vi "Polar Graph Drawer.vi"(8 "error in":errorcluster, 10 "Plot Right":dbl[](array[numeric]), 11 "Plot Left":dbl[](array[numeric])) -> (0 "error out":errorcluster, 3 "Polar Graph":cluster{dbl[], dbl[]}[](graph))   [LabVIEW 2025]
uses:
  <vilib>/Analysis/baseanly.llb/Mean (DBL).vi
  <vilib>/Analysis/NI_AALBase.lvlib
  <vilib>/gmath/NI_Gmath.lvlib
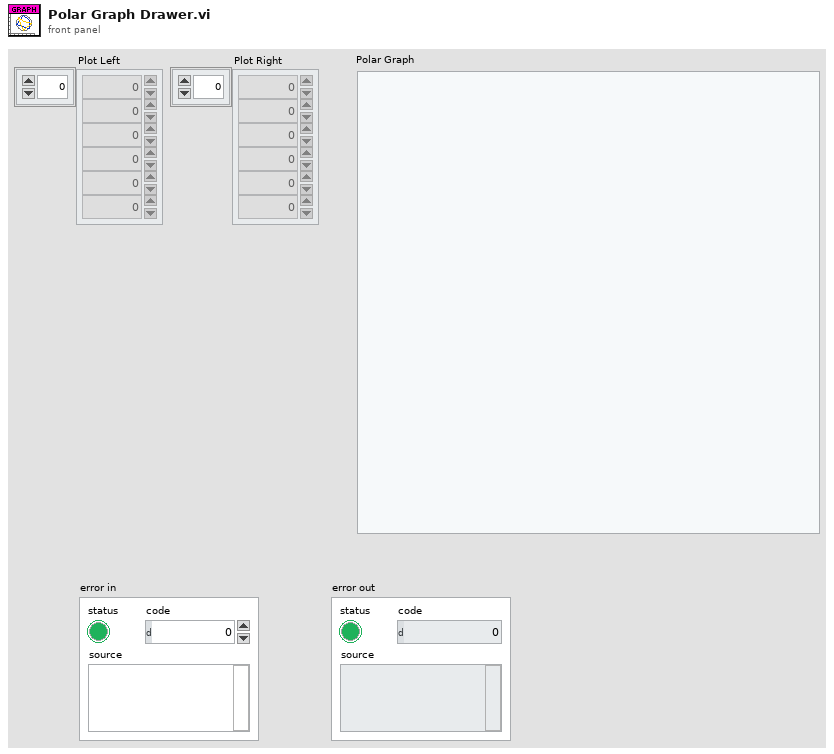
[diagram p1: front panel]
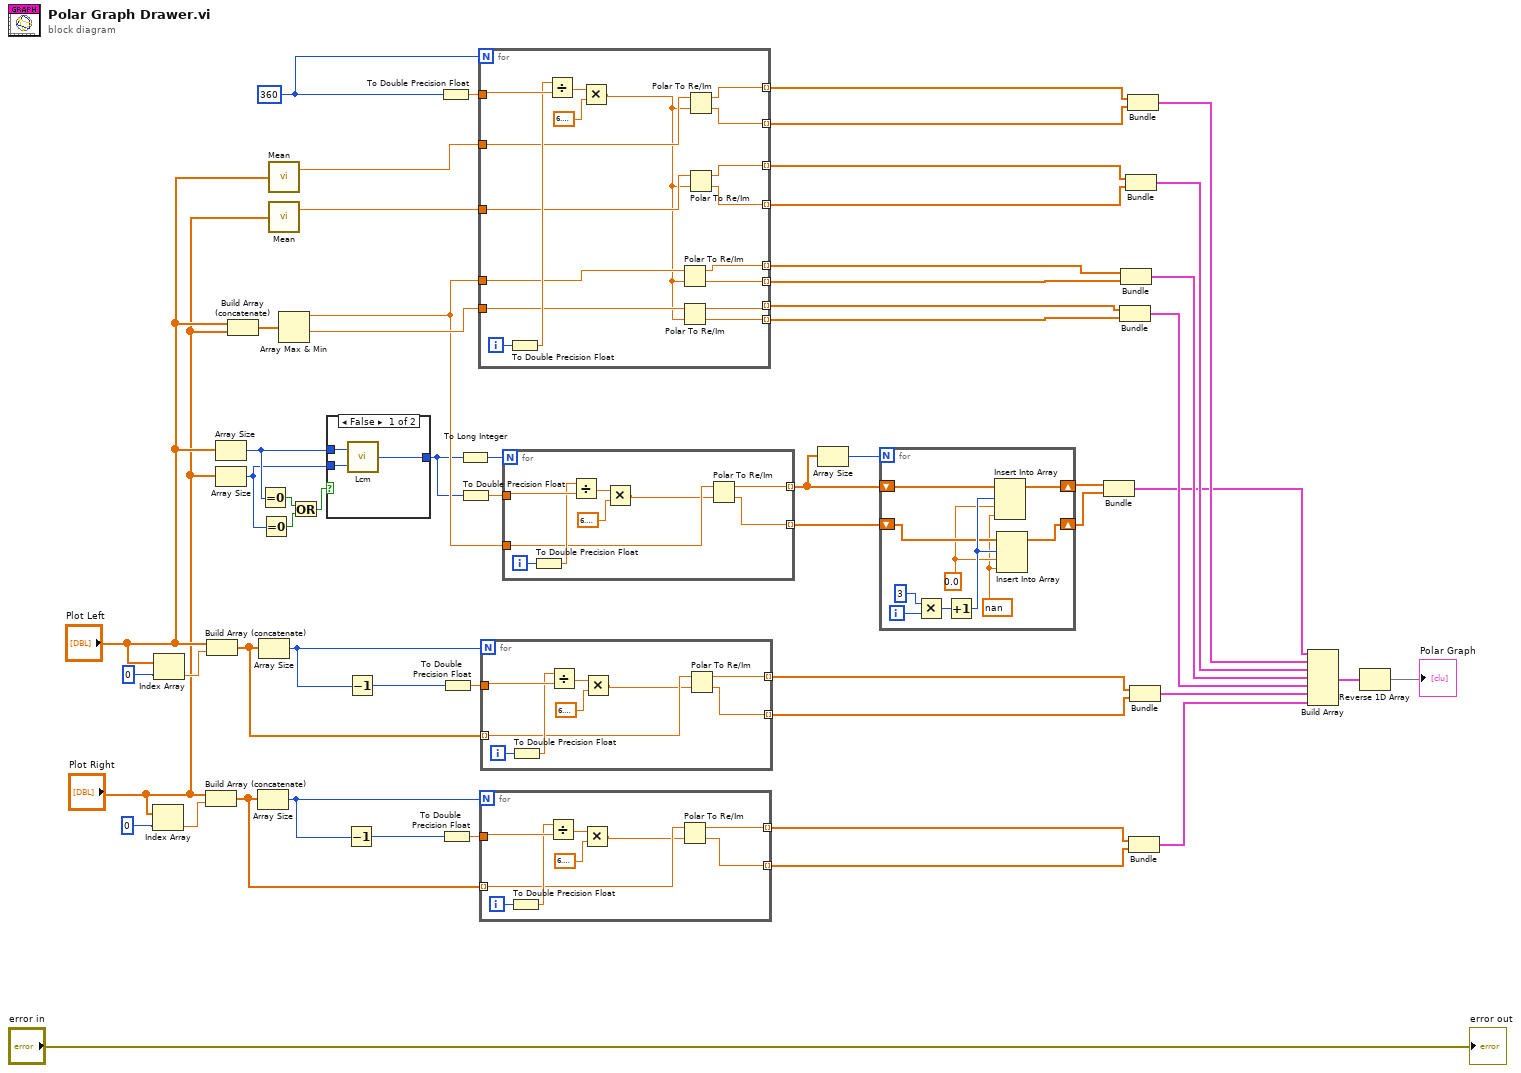
[diagram p0: block diagram]
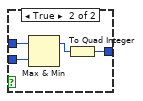
[diagram p2: hidden frame]
diagram:
  w35 = 360
  n1 = Index Array(array="Plot Right", index=0) -> (element=w44:dbl)
  n2 = Index Array(array="Plot Left", index=0) -> (element=w53:dbl)
  n3 = Build Array (concatenate)("Plot Right", w44) -> (w42:dbl[])
  n4 = Build Array (concatenate)("Plot Left", w53) -> (w51:dbl[])
  n5 = Array Size(array="Plot Left") -> (size(s)=w5:i32)
  n6 = Array Size(array="Plot Right") -> (size(s)=w4:i32)
  n7 = Build Array (concatenate)("Plot Left", "Plot Right") -> (w32:dbl[])
  n8 = Array Size(array=w42) -> (size(s)=w40:i32)
  n9 = Array Size(array=w51) -> (size(s)=w49:i32)
  n10 = Equal To 0?(x=w5) -> (x = 0?=w3:bool)
  n11 = Equal To 0?(x=w4) -> (x = 0?=w2:bool)
  n12 = call-poly <vilib>:"Mean.vi"("X"="Plot Left") -> ("mean"=w19:dbl)  [unwired: 1 out]
  n13 = call-poly <vilib>:"Mean.vi"("X"="Plot Right") -> ("mean"=w20:dbl)  [unwired: 1 out]
  n14 = Array Max & Min(array=w32) -> (max value=w15:dbl, min value=w29:dbl)  [unwired: 2 out]
  n15 = Or(x=w3, y=w2) -> (x .or. y?=w1:bool)
  n16 = case shown="False" w1 {
    tunnel: [w59 w61] -> w12
    tunnel: w5 -> [w58 w63]
    tunnel: w4 -> [w57 w62]
    frame False {
      n17 = call <vilib>:"Lcm.vi"("y"=w57, "x"=w58) -> ("lcm(x,y)"=w59:i64)
    }
    frame True {
      n18 = Max & Min(x=w63, y=w62) -> (max(x,y)=w60:i32)  [unwired: 1 out]
      n19 = To Quad Integer(1:w60) -> (0:w61:i64)
    }
  }
  n20 = Decrement(x=w40) -> (x-1=w41:i32)
  n21 = Decrement(x=w49) -> (x-1=w50:i32)
  n22 = To Double Precision Float(number=w35) -> (double precision float=w38:dbl)
  n23 = To Double Precision Float(number=w41) -> (double precision float=w47:dbl)
  n24 = To Double Precision Float(number=w50) -> (double precision float=w56:dbl)
  n25 = To Long Integer(number=w12) -> (32bit integer=w14:i32)
  n26 = To Double Precision Float(number=w12) -> (double precision float=w13:dbl)
  n27 = for {
    N: w35 -> [_]
    tunnel: w38 -> [w78]
    tunnel: [w71] -> w36 mode=indexing
    tunnel: [w72] -> w37 mode=indexing
    tunnel: w19 -> [w73]
    tunnel: [w76] -> w34 mode=indexing
    tunnel: [w75] -> w33 mode=indexing
    tunnel: w20 -> [w74]
    tunnel: w15 -> [w69]
    tunnel: w29 -> [w70]
    tunnel: [w67] -> w27 mode=indexing
    tunnel: [w66] -> w28 mode=indexing
    tunnel: [w65] -> w26 mode=indexing
    tunnel: [w64] -> w25 mode=indexing
    i -> [w81]
    n28 = To Double Precision Float(number=w81) -> (double precision float=w77:dbl)
    n29 = Divide(x=w77, y=w78) -> (x/y=w80:dbl)
    n30 = Multiply(x=w80, y=6.283185307179586) -> (x*y=w68:dbl)
    n31 = Polar To Re/Im(2:w68, 3:w69) -> (0:w67:dbl, 1:w66:dbl)
    n32 = Polar To Re/Im(2:w68, 3:w70) -> (0:w64:dbl, 1:w65:dbl)
    n33 = Polar To Re/Im(2:w68, 3:w73) -> (0:w71:dbl, 1:w72:dbl)
    n34 = Polar To Re/Im(2:w68, 3:w74) -> (0:w75:dbl, 1:w76:dbl)
  }
  n35 = for {
    N: w40 -> [_]
    tunnel: w47 -> [w87]
    tunnel: [w84] -> w45 mode=indexing
    tunnel: [w85] -> w46 mode=indexing
    tunnel: w42 -> [w83] mode=indexing
    i -> [w90]
    n36 = To Double Precision Float(number=w90) -> (double precision float=w86:dbl)
    n37 = Divide(x=w86, y=w87) -> (x/y=w89:dbl)
    n38 = Multiply(x=w89, y=6.283185307179586) -> (x*y=w82:dbl)
    n39 = Polar To Re/Im(2:w82, 3:w83) -> (0:w84:dbl, 1:w85:dbl)
  }
  n40 = for {
    N: w49 -> [_]
    tunnel: w56 -> [w96]
    tunnel: [w91] -> w54 mode=indexing
    tunnel: [w92] -> w55 mode=indexing
    tunnel: w51 -> [w94] mode=indexing
    i -> [w99]
    n41 = To Double Precision Float(number=w99) -> (double precision float=w95:dbl)
    n42 = Divide(x=w95, y=w96) -> (x/y=w98:dbl)
    n43 = Multiply(x=w98, y=6.283185307179586) -> (x*y=w93:dbl)
    n44 = Polar To Re/Im(2:w93, 3:w94) -> (0:w91:dbl, 1:w92:dbl)
  }
  n45 = for {
    N: w14 -> [_]
    tunnel: w13 -> [w105]
    tunnel: [w100] -> w11 mode=indexing
    tunnel: [w101] -> w10 mode=indexing
    tunnel: w15 -> [w103]
    i -> [w108]
    n46 = To Double Precision Float(number=w108) -> (double precision float=w104:dbl)
    n47 = Divide(x=w104, y=w105) -> (x/y=w107:dbl)
    n48 = Multiply(x=w107, y=6.283185307179586) -> (x*y=w102:dbl)
    n49 = Polar To Re/Im(2:w102, 3:w103) -> (0:w100:dbl, 1:w101:dbl)
  }
  n50 = Array Size(array=w10) -> (size(s)=w9:i32)
  n51 = for {
    N: w9 -> [_]
    shift-right: [w111] -> w7
    shift-left: w10 -> [w118]
    shift-right: [w112] -> w8
    shift-left: w11 -> [w113]
    i -> [w117]
    w109 = nan
    w110 = 0.0 ("new element/subarray")
    n52 = Multiply(x=3, y=w117) -> (x*y=w115:i32)
    n53 = Increment(x=w115) -> (x+1=w114:i32)
    n54 = Insert Into Array(array=w118, index=w114, new element #1=w110, new element #2=w109) -> (w111:dbl[])
    n55 = Insert Into Array(array=w113, index=w114, new element #1=w110, new element #2=w109) -> (w112:dbl[])
  }
  n56 = Bundle(w7, w8) -> (w6:cluster{dbl[], dbl[]})  [unwired: 1 in]
  n57 = Bundle(w26, w25) -> (w24:cluster{dbl[], dbl[]})  [unwired: 1 in]
  n58 = Bundle(w28, w27) -> (w23:cluster{dbl[], dbl[]})  [unwired: 1 in]
  n59 = Bundle(w34, w33) -> (w31:cluster{dbl[], dbl[]})  [unwired: 1 in]
  n60 = Bundle(w37, w36) -> (w30:cluster{dbl[], dbl[]})  [unwired: 1 in]
  n61 = Bundle(w46, w45) -> (w39:cluster{dbl[], dbl[]})  [unwired: 1 in]
  n62 = Bundle(w55, w54) -> (w48:cluster{dbl[], dbl[]})  [unwired: 1 in]
  n63 = Build Array(w6, w30, w31, w23, w24, w48, w39) -> (w22:cluster{dbl[], dbl[]}[])
  n64 = Reverse 1D Array(array=w22) -> (reversed array=→"Polar Graph":cluster{dbl[], dbl[]}[])
  "error out" <- "error in"
